vi "Calibration Helper2.vi"(7 "Std Devs":cluster{"H":dbl, "S":dbl, "V":dbl}={"H"=4.0, "S"=6.0, "V"=6.0}, 8 "Color Mode":u16(ring)=2 items=["RGB", "HSL", "HSV", "HSI", "CIE L*a*b*", "CIE XYZ"], 10 "Image":T1, 11 "Image Ctl Refnum":refnum<vi>) -> (2 "Changed":bool, 3 "output color":T2)   [LabVIEW 2025]
doc: "Use the ROI (region of interest) to mask the image and compute a histogram of the indicated region. This provides the average H, S, and V values as well as the\nstandard deviation of each. It then calculates the initial upper and lower values we want to use for the threshold, and ensure that they are between 0 and 255. Hue, or the 0'th item is\na circular coordinate, so we sometimes flip the upper and lower when the computed value wraps past zero. The other values are linear and are simply clamped. This statistical approach is a reasonable approach when the ROI makes sense, but it is often useful to adjust the high/low values after the auto-calibration."
uses:
  <vilib>/vision/Image Controls.llb/IMAQ Image.ctl
  <vilib>/vision/NI_Vision_Development_Module.lvlib
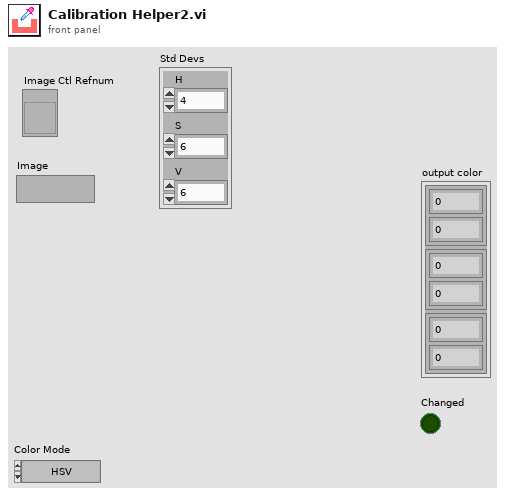
[diagram p1: front panel]
types:
  T1 = typedef "IMAQ Image.ctl" = refnum<image>
  T2 = cluster{cluster{"Lower":dbl, "Upper":dbl}, cluster{"Lower":dbl, "Upper":dbl}, cluster{"Lower":dbl, "Upper":dbl}}
  T3 = typedef "Image Type" = u32
  T4 = cluster{"Global Rectangle":i32[], "Contours":cluster{"Contour Type":u32, "ROI Type":u32, "Points":i32[]}[]}
  T5 = cluster{"histogram":u32[], "Minimal Value":sgl, "Maximal Value":sgl, "Starting Value":sgl, "Interval Width":sgl, "Mean Value":sgl, "Standard  Variation":sgl, "Area (pixels)":i32}
  T6 = cluster{"histogram":u32[], "Minimal Value":sgl, "Maximal Value":sgl, "Starting Value":sgl, "Interval Width":sgl, "Mean Value":sgl, "Standard  Variation":sgl, "Area (pixels)":i32}[]
  T7 = cluster{"[0]":cluster{dbl, dbl}, "[1]":cluster{dbl, dbl}, "[2]":cluster{dbl, dbl}}
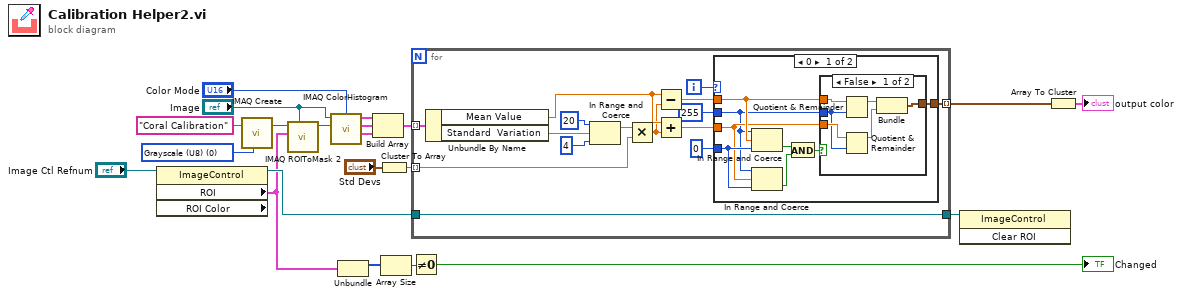
[diagram p0: block diagram]
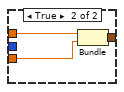
[diagram p2: hidden frame]
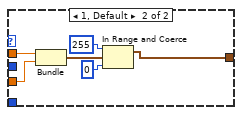
[diagram p3: hidden frame]
diagram:
  w18 = T3 0 items=["Grayscale (U8)", "Grayscale (I16)", "Grayscale (SGL)", "Complex (CSG)", "RGB (U32)", "HSL (U32)", "RGB (U64)", "Grayscale (U16)"] ("Image Type")
  n1 = property on="Property Node" class="ImageControl" props=["ROI", "ROI Color"](reference="Image Ctl Refnum") -> (reference out=w4:refnum<vi>, "ROI"=w3:T4)  [unwired: 1 in, 2 out]
  n2 = call "IMAQ Create"("Image Name"="Coral Calibration", "Image Type"=w18) -> ("New Image"=w15:T1)  [unwired: 3 in, 1 out]
  n3 = call "IMAQ ROIToMask 2"("Image Model"="Image", "ROI Descriptor"=w3, "Image"=w15) -> ("Image Out"=w16:T1)  [unwired: 6 in, 2 out]
  n4 = call "IMAQ ColorHistogram"("Color Mode"="Color Mode", "Image Src"="Image", "Image Mask"=w16) -> ("Red or Hue or X or L* Histogram Report"=w11:T5, "Green or Sat or Y or a* Histogram Report"=w10:T5, "Blue or Luma or Val or Inten or Z or b* Histogram Report"=w9:T5)  [unwired: 3 in, 1 out]
  n5 = Unbundle(w3) -> ("Global Rectangle"=w2:i32[])  [unwired: 1 out]
  n6 = Build Array(w11, w10, w9) -> (w7:T6)
  n7 = Cluster To Array(cluster="Std Devs") -> (array=w8:dbl[])
  n8 = Array Size(array=w2) -> (size(s)=w1:i32)
  n9 = Not Equal To 0?(x=w1) -> (x != 0?=→"Changed":bool)
  n10 = for {
    tunnel: w8 -> [w32] mode=indexing
    tunnel: w7 -> [w36] mode=indexing
    tunnel: [w27] -> w6 mode=indexing
    tunnel: [w22] -> w5
    tunnel: w4 -> [w22]
    i -> [w25]
    n11 = Unbundle By Name(w36) -> ("Mean Value"=w30:sgl, "Standard  Variation"=w33:sgl)
    n12 = In Range and Coerce(upper limit=20, x=w33, lower limit=4) -> (coerced(x)=w31:sgl)  [unwired: 1 out]
    n13 = Multiply(x=w31, y=w32) -> (x*y=w26:dbl)
    n14 = Subtract(x=w30, y=w26) -> (x-y=w29:dbl)
    n15 = Add(x=w30, y=w26) -> (x+y=w28:dbl)
    n16 = case shown="0" w25 {
      tunnel: w29 -> [w39 w56]
      tunnel: w28 -> [w38 w55]
      tunnel: [w41 w54] -> w27
      tunnel: 255 -> [w37 _]
      tunnel: 0 -> [w40 _]
      frame 0 {
        n17 = In Range and Coerce(upper limit=w37, x=w39, lower limit=w40) -> (In Range?=w43:bool)  [unwired: 1 out]
        n18 = In Range and Coerce(upper limit=w37, x=w38, lower limit=w40) -> (In Range?=w42:bool)  [unwired: 1 out]
        n19 = And(x=w43, y=w42) -> (x .and. y?=w44:bool)
        n20 = case shown="False" w44 {
          tunnel: [w47 w53] -> w41
          tunnel: w39 -> [w50 w51]
          tunnel: w38 -> [w49 w52]
          tunnel: w37 -> [w48 _]
          frame False {
            n21 = Quotient & Remainder(x=w50, y=w48) -> (x-y*floor(x/y)=w45:dbl)  [unwired: 1 out]
            n22 = Quotient & Remainder(x=w49, y=w48) -> (x-y*floor(x/y)=w46:dbl)  [unwired: 1 out]
            n23 = Bundle(w45, w46) -> (w47:cluster{dbl, dbl})  [unwired: 1 in]
          }
          frame True {
            n24 = Bundle(w51, w52) -> (w53:cluster{dbl, dbl})  [unwired: 1 in]
          }
        }
      }
      frame 1, Default {
        n25 = Bundle(w56, w55) -> (w59:cluster{dbl, dbl})  [unwired: 1 in]
        n26 = In Range and Coerce(upper limit=255, x=w59, lower limit=0) -> (coerced(x)=w54:cluster{dbl, dbl})  [unwired: 1 out]
      }
    }
  }
  n27 = invoke on="Invoke Node" class="ImageControl" method="Clear ROI"(reference=w5) -> ()  [unwired: 2 in, 3 out]
  n28 = Array To Cluster(array=w6) -> (cluster=→"output color":T7)
